vi "whilefor.vi"() -> ()   [LabVIEW 2022 SP3]
panel:
  out "current value of iterator":dbl
  out "end of loop":bool
  in  "stop":bool
  in  "Limit":i32 format="%#.0g"
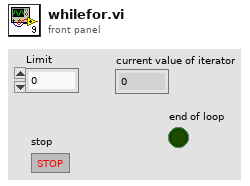
[diagram p1: front panel]
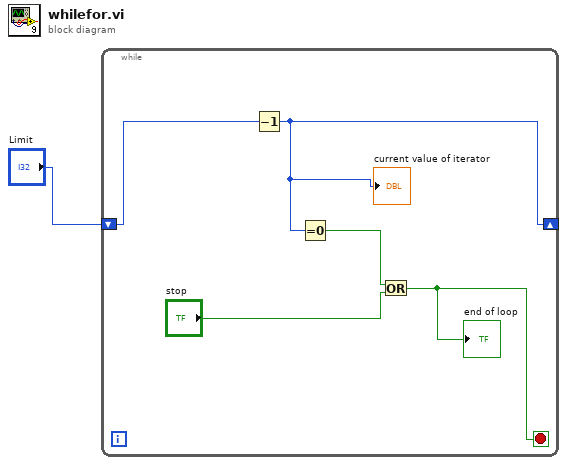
[diagram p0: block diagram]
diagram:
  n1 = while {
    shift-right: [w2] -> _
    shift-left: "Limit" -> [w6]
    stop <- w3 stop-if-true
    n2 = Decrement(x=w6) -> (x-1=w2:i32)
    "current value of iterator" <- w2
    n3 = Equal To 0?(x=w2) -> (x = 0?=w4:bool)
    n4 = Or(x=w4, y="stop") -> (x .or. y?=w3:bool)
    "end of loop" <- w3
  }
